vi "Recieve command.vi"(0 "reference in":refnum<class "NS slave.lvclass">, 11 "error in (no error)":errorcluster, 13 "timeout ms (100)":i32=100) -> (4 "reference out":refnum<class "NS slave.lvclass">, 6 "message":string, 8 "parameters":string, 10 "data":variant, 14 "timed out?":bool, 15 "error out":errorcluster)   [LabVIEW 2019, in "CommandResponse communication.lvlib" / "NS slave.lvclass"]
doc: "Recives command as message + variant data"
uses:
  NS slave.lvclass
  C:/Barkhausen mmWave radar/Development/LV/Barkhausen mmWave hardware control/Host/Intertarget communication/CR slave_class/CR slave.lvclass
  ITC command.ctl
  <resource>/objmgr/ni.dex.rc
  CommandResponse communication.lvlib
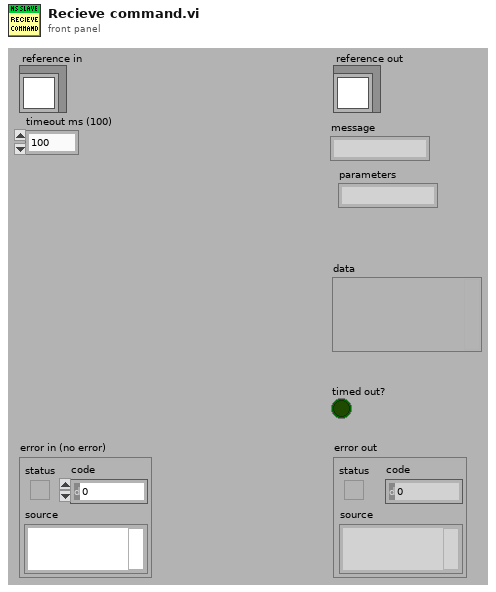
[diagram p1: front panel]
types:
  T1 = typedef "CommandResponse communication.lvlib/NS slave.lvclass/ObjectAttributesRef.ctl" = refnum<data-value>
  T2 = typedef "CommandResponse communication.lvlib/NS slave.lvclass/ObjectAttributes.ctl" = cluster{"connected":bool, "stop":bool, "ID":string, "command rd":refnum<k21>, "response wr":refnum<k21>, "data wr":refnum<k21>}
  T3 = typedef "CommandResponse communication.lvlib/ITC command.ctl" = cluster{"message":string, "parameters":string, "data":variant}
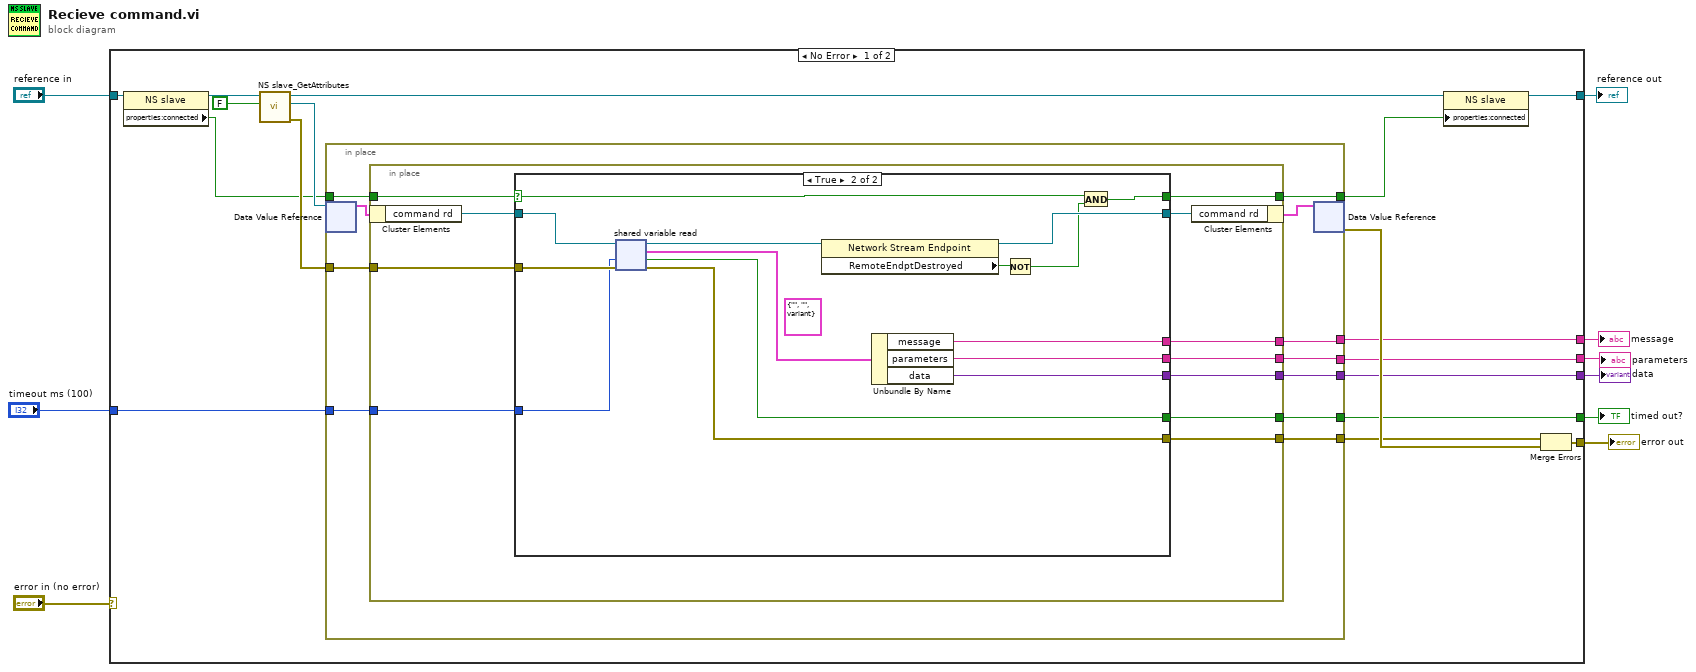
[diagram p0: block diagram]
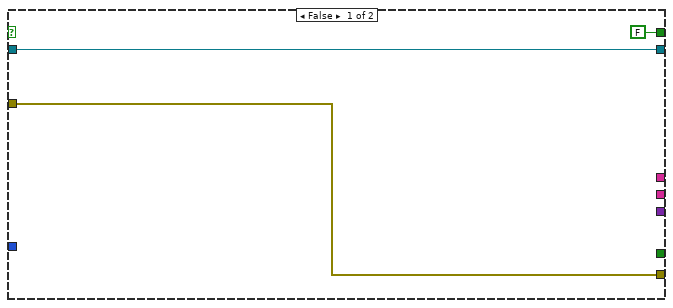
[diagram p2: hidden frame]
diagram:
  n1 = case shown="No Error" "error in (no error)" {
    selector: "error in (no error)" -> [_ w68]
    tunnel: [w26 w68] -> w8
    tunnel: [w13 w67] -> w6
    tunnel: "reference in" -> [w23 w67]
    tunnel: "timeout ms (100)" -> [w18 _]
    tunnel: [w17 _] -> w4
    tunnel: [w16 _] -> w3
    tunnel: [w15 _] -> w2
    tunnel: [w14 _] -> w1
    frame No Error {
      n2 = property class="NS slave"(reference=w23) -> (reference out=w12:refnum<class "NS slave.lvclass">, "properties:connected"=w11:bool)  [unwired: 1 in, 1 out]
      n3 = call "NS slave_GetAttributes.vi"("return data? (T)"=FALSE, "reference in"=w12) -> ("error out"=w19:errorcluster, "attributes ref"=w20:T1, "reference out"=w21:refnum<class "NS slave.lvclass">)  [unwired: 6 in, 1 out]
      n4 = in-place {
        in-place-border: [w34] -> w24
        in-place-border: w19 -> [w35]
        in-place-border: w18 -> [w33]
        in-place-border: [w32] -> w16
        in-place-border: [w31] -> w17
        in-place-border: [w30] -> w15
        in-place-border: [w29] -> w14
        in-place-border: w11 -> [w28]
        in-place-border: [w27] -> w10
        n5 = in-place-dvr #1(w20) -> (w36:T2)  [unwired: 1 out]
        n6 = in-place {
          in-place-border: w35 -> [w46]
          in-place-border: [w45] -> w34
          in-place-border: w33 -> [w44]
          in-place-border: [w43] -> w31
          in-place-border: [w42] -> w32
          in-place-border: [w41] -> w30
          in-place-border: [w40] -> w29
          in-place-border: w28 -> [w39]
          in-place-border: [w38] -> w27
          n7 = in-place-cluster #2(w36) -> ("command rd"=w48:refnum<k21>)
          n8 = case shown="True" w39 {
            selector: w39 -> [_ w64]
            tunnel: w48 -> [w51 w66]
            tunnel: [w51 w56] -> w47
            tunnel: w46 -> [w50 w65]
            tunnel: [w50 w62] -> w45
            tunnel: [FALSE w54] -> w38
            tunnel: w44 -> [_ w61]
            tunnel: [_ w59] -> w43
            tunnel: [_ w58] -> w42
            tunnel: [_ w57] -> w41
            tunnel: [_ w52] -> w40
            frame False {
            }
            frame True {
              (unwired) T3 {"message"="", "parameters"="", "data"=variant} ("data out")
              n9 = shared-variable-read(w66, w65, w61) -> (w63:refnum<k21>, w62:errorcluster, w57:bool, w60:T3)
              n10 = property class="Network Stream Endpoint"(reference=w63) -> (reference out=w56:refnum<k21>, "RemoteEndptDestroyed"=w55:bool)  [unwired: 1 in, 1 out]
              n11 = Unbundle By Name(w60) -> ("message"=w59:string, "parameters"=w58:string, "data"=w52:variant)
              n12 = Not(x=w55) -> (.not. x?=w53:bool)
              n13 = And(x=w64, y=w53) -> (x .and. y?=w54:bool)
            }
          }
          n14 = in-place-cluster #2("command rd"=w47) -> (w37:T2)
        }
        n15 = in-place-dvr #1(w37) -> (w25:errorcluster)  [unwired: 1 out]
      }
      n16 = property class="NS slave"(reference=w21, "properties:connected"=w10) -> (reference out=w13:refnum<class "NS slave.lvclass">)  [unwired: 1 in, 1 out]
      n17 = Merge Errors(w24, w25) -> (w26:errorcluster)
    }
    frame Error {
    }
  }
  "error out" <- w8
  "reference out" <- w6
  "message" <- w4
  "parameters" <- w3
  "timed out?" <- w2
  "data" <- w1
